vi "Finish.vi"(8 "error in (no error)":errorcluster, 11 "TalonSRX in":refnum<class "TalonSRX.lvclass">) -> (0 "error out":errorcluster, 3 "TalonSRX out":refnum<class "TalonSRX.lvclass">)   [LabVIEW 2019, in "Drive.lvlib" / "TalonSRX.lvclass"]
uses:
  TalonSRX.lvclass
  CTRE Drive.lvclass
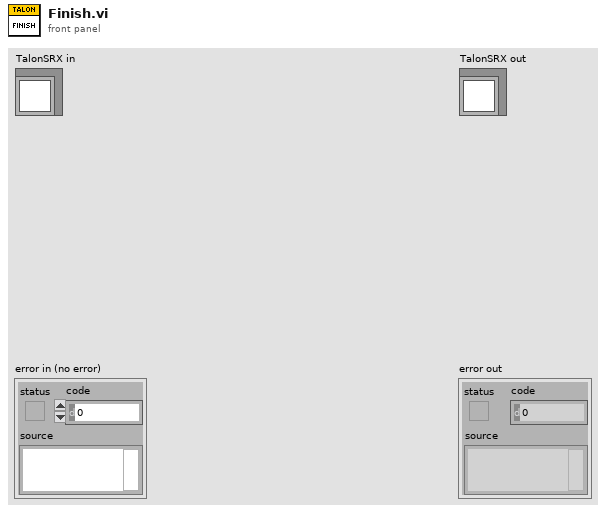
[diagram p1: front panel]
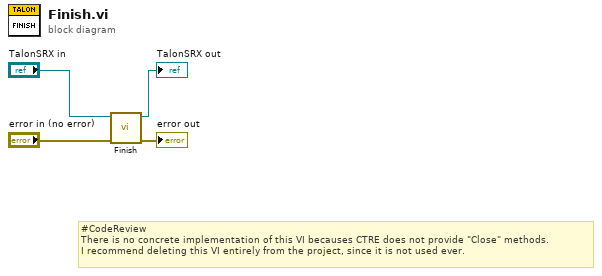
[diagram p0: block diagram]
diagram:
  # "#CodeReview\nThere is no concrete implementation of this VI becauses CTRE does not provide \"Close\" methods.\nI recommend deleting this VI entirely from the project, since it is not used ever."
  n1 = call-parent "Finish.vi"("error in (no error)"="error in (no error)", "Tank Drive in"="TalonSRX in") -> ("error out"=→"error out":errorcluster, "Tank Drive out"=→"TalonSRX out":refnum<class "TalonSRX.lvclass">)  [unwired: 8 in]
